vi "Generador_Funciones.vi"() -> ()   [LabVIEW 2015]
panel:
  in  "Offset":dbl(knob) scale=0.0..10.0
  in  "Amplitud":dbl(knob) scale=0.0..10.0
  out "Waveform Chart":dbl(graph)
  in  "Enum":T1(ring)
  out "Numeric Control":dbl
  in  "Stop Button":bool
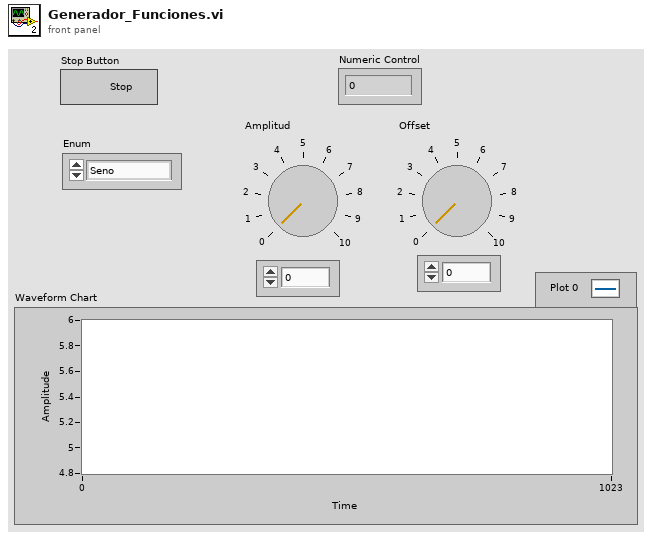
[diagram p1: front panel]
types:
  T1 = enum16{"Seno", "Triangular", "Diente de Sierra", "Pulso", "Secante", "Tangente", "DC", "GND"}
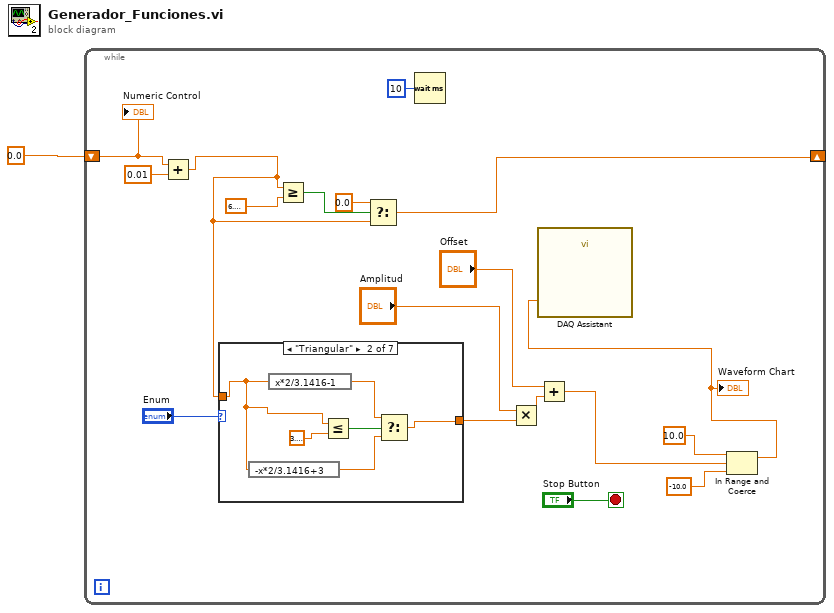
[diagram p0: block diagram]
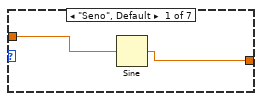
[diagram p2: hidden frame]
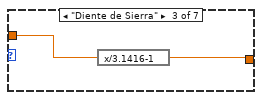
[diagram p3: hidden frame]
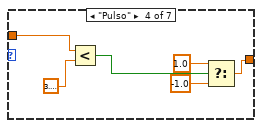
[diagram p4: hidden frame]
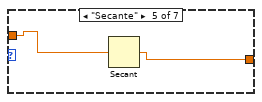
[diagram p5: hidden frame]
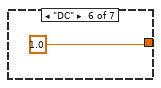
[diagram p6: hidden frame]
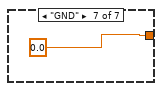
[diagram p7: hidden frame]
diagram:
  n1 = while {
    shift-right: [w12] -> _
    shift-left: 0.0 -> [w19]
    stop <- "Stop Button" stop-if-true
    n2 = Add(x=w19, y=0.01) -> (x+y=w10:dbl)
    n3 = case shown="\"Triangular\"" "Enum" {
      tunnel: w10 -> [w21 w27 w29 w34 w37 _ _]
      tunnel: [w20 w24 w28 w30 w36 1.0 ("y") 0.0 ("y")] -> w9
      frame "Seno", Default {
        n4 = Sine(x=w21) -> (sin(x)=w20:dbl)
      }
      frame "Triangular" {
        n5 = expression code="-x*2/3.1416+3"(w27) -> (w23:dbl)
        n6 = expression code="x*2/3.1416-1"(w27) -> (w22:dbl)
        n7 = Less Or Equal?(x=w27, y=3.141592653589793) -> (x <= y?=w25:bool)
        n8 = Select(t=w22, s=w25, f=w23) -> (s? t:f=w24:dbl)
      }
      frame "Diente de Sierra" {
        n9 = expression code="x/3.1416-1"(w29) -> (w28:dbl)
      }
      frame "Pulso" {
        n10 = Less?(x=w34, y=3.141592653589793) -> (x < y?=w35:bool)
        n11 = Select(t=1.0, s=w35, f=-1.0) -> (s? t:f=w30:dbl)
      }
      frame "Secante" {
        n12 = Secant(1:w37) -> (0:w36:dbl)
      }
      frame "DC" {
      }
      frame "GND" {
      }
    }
    n13 = Greater Or Equal?(x=w10, y=6.283185307179586) -> (x >= y?=w14:bool)
    n14 = Select(t=0.0, s=w14, f=w10) -> (s? t:f=w12:dbl)
    n15 = Wait (ms)(milliseconds to wait=u32 10) -> ()  [unwired: 1 out]
    n16 = Multiply(x="Amplitud", y=w9) -> (x*y=w7:dbl)
    n17 = Add(x="Offset", y=w7) -> (x+y=w3:dbl)
    n18 = In Range and Coerce(upper limit=10.0, x=w3, lower limit=-10.0) -> (coerced(x)=w2:dbl)  [unwired: 1 out]
    "Waveform Chart" <- w2
    n19 = call "DAQ Assistant"("data"=w2) -> ()  [unwired: 17 in, 2 out]
    "Numeric Control" <- w19
  }
